vi "_Update Connection.vi"(8 "error in (no error)":errorcluster, 9 "Info":T1, 10 "Data in":T3) -> (0 "error out":errorcluster, 2 "Data":T3)   [LabVIEW 2020, in "Vecto.lvlib" / "VectoInfo.lvclass"]
uses:
  VectoInfo.lvclass
  VectoInfo.lvclass/VectoInfo.ctl
  <vilib>/Utility/miscctls.llb/LVMapReplaceAction.ctl
  f2202518-d15a-43f6-8f49-198556fefdba.vi
  76580e86-6d32-45c5-a73e-d65301a86c10.vi
  6d027098-dc54-4dc8-bb79-6d6b344b4b44.vi
  da43e2c0-df91-4218-9e50-031a37b01e1a.vi
  fa79f708-6420-48c4-aeb2-96318dfe20dd.vi
  7961e0f9-2531-422f-8d50-442907a070aa.vi
  Connection Type.ctl
  Vecto.lvlib
  Connection Info.ctl
  Vecto Info.ctl
  Loop Data.ctl
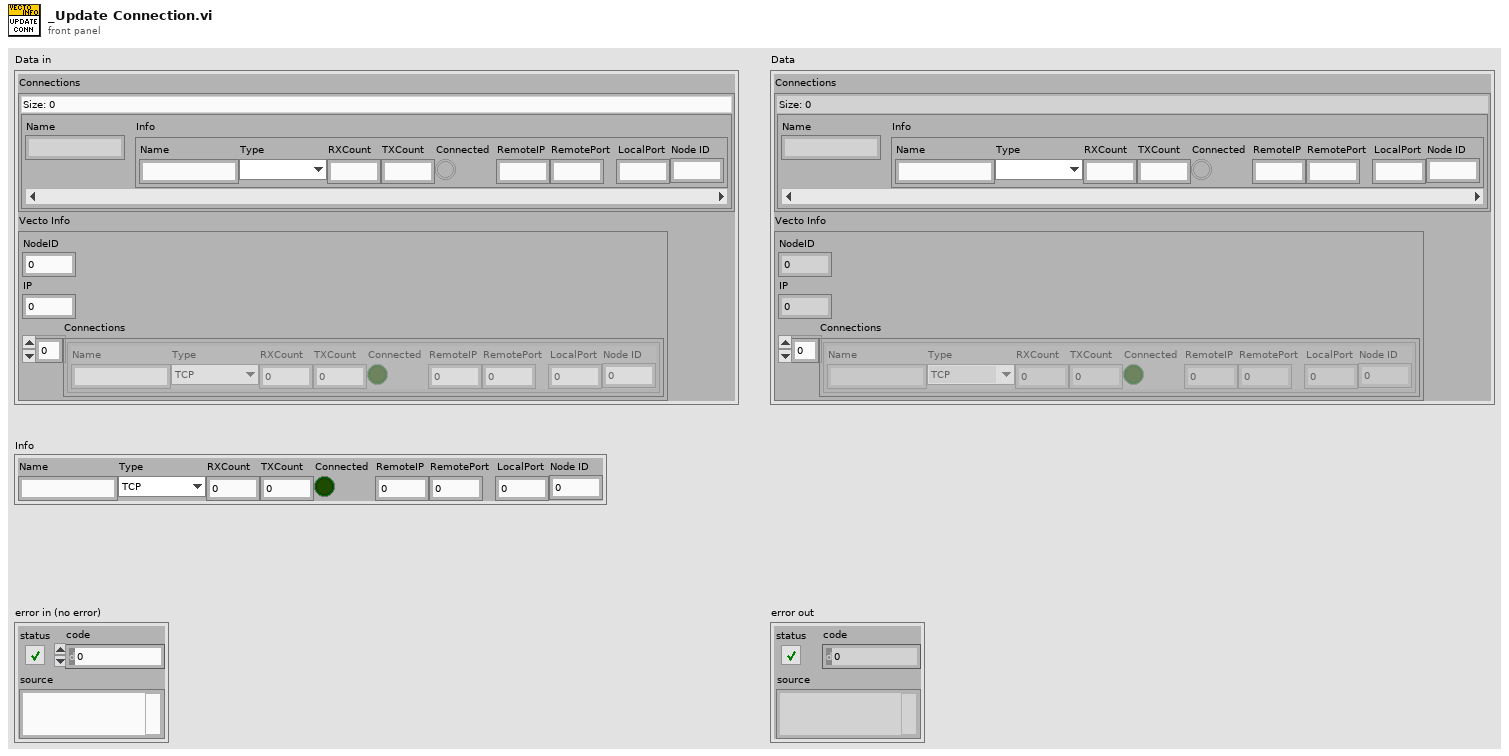
[diagram p1: front panel]
types:
  T1 = typedef "Vecto.lvlib/Connection Info.ctl" = cluster{"Name":string, "Type":T2, "RXCount":i32, "TXCount":i32, "Connected":bool, "RemoteIP":u32, "RemotePort":u16, "LocalPort":u16, "Node ID":u32}
  T2 = typedef "Vecto.lvlib/Connection Type.ctl" = enum16{"TCP", "Telemetry", "Discovery", "HTTP"}
  T3 = typedef "Vecto.lvlib/VectoInfo.lvclass/Loop Data.ctl" = cluster{"Connections":map{string, T1}, "Vecto Info":T4}
  T4 = typedef "Vecto.lvlib/Vecto Info.ctl" = cluster{"NodeID":i32, "IP":u32, "Connections":T1[]}
  T5 = typedef "LVMapReplaceAction.ctl" = enum32{"Modify Entry only if found", "Add or Modify Entry", "Delete Entry"}
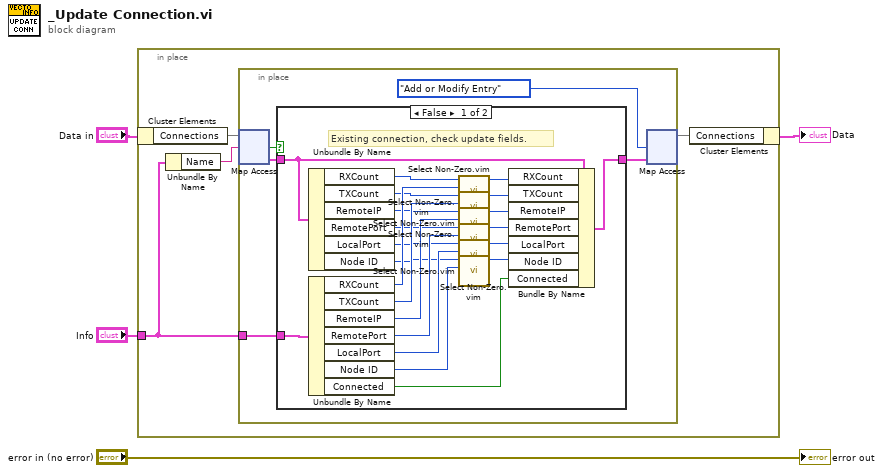
[diagram p0: block diagram]
diagram:
  n1 = in-place {
    in-place-border: "Info" -> [w5]
    n2 = in-place-cluster #1("Data in") -> ("Connections"=w8:map{string, T1})
    n3 = Unbundle By Name(w5) -> ("Name"=w6:string)
    n4 = in-place {
      in-place-border: w5 -> [w9]
      n5 = in-place-map #2(w8, w6) -> (w12:T1, w11:bool)  [unwired: 1 in]
      n6 = case shown="False" w11 {
        tunnel: w12 -> [w34 _]
        tunnel: [w33 w36] -> w10
        tunnel: w9 -> [w35 w36]
        frame False {
          # "Existing connection, check update fields."
          n7 = Unbundle By Name(w34) -> ("RXCount"=w32:i32, "TXCount"=w29:i32, "RemoteIP"=w27:u32, "RemotePort"=w25:u16, "LocalPort"=w23:u16, "Node ID"=w21:u32)
          n8 = Unbundle By Name(w35) -> ("RXCount"=w31:i32, "TXCount"=w28:i32, "RemoteIP"=w26:u32, "RemotePort"=w24:u16, "LocalPort"=w22:u16, "Node ID"=w20:u32, "Connected"=w14:bool)
          n9 = call "Select Non-Zero.vim"("B"=w31, "A"=w32) -> ("Non-Zero"=w30:i32)  [unwired: 9 in]
          n10 = call "Select Non-Zero.vim"("B"=w28, "A"=w29) -> ("Non-Zero"=w19:i32)  [unwired: 9 in]
          n11 = call "Select Non-Zero.vim"("B"=w26, "A"=w27) -> ("Non-Zero"=w18:u32)  [unwired: 9 in]
          n12 = call "Select Non-Zero.vim"("B"=w24, "A"=w25) -> ("Non-Zero"=w17:u16)  [unwired: 9 in]
          n13 = call "Select Non-Zero.vim"("B"=w22, "A"=w23) -> ("Non-Zero"=w16:u16)  [unwired: 9 in]
          n14 = call "Select Non-Zero.vim"("B"=w20, "A"=w21) -> ("Non-Zero"=w15:u32)  [unwired: 9 in]
          n15 = Bundle By Name(cluster=w34, "RXCount"=w30, "TXCount"=w19, "RemoteIP"=w18, "RemotePort"=w17, "LocalPort"=w16, "Node ID"=w15, "Connected"=w14) -> (w33:T1)
        }
        frame True {
          # "New connection, just use provided info"
        }
      }
      n16 = in-place-map #2(w10, LVMapReplaceAction."Add or Modify Entry" ("action")) -> (w7:map{string, T1})  [unwired: 2 out]
    }
    n17 = in-place-cluster #1("Connections"=w7) -> (→"Data":T3)
  }
  "error out" <- "error in (no error)"
